vi "Get Switch.vi"(8 "error in (no error)":errorcluster, 10 "switch name":string="A", 11 "MC switch refnum in":refnum<k24>) -> (0 "error out":errorcluster, 2 "state":bool, 3 "MC switch refnum out":refnum<k24>)   [LabVIEW 2019, in "Minicircuit RF Switch Box.lvlib"]
doc: "This function get an individual SPDT state within the switch matrix. The switches are designated A to H, as labeled on the front of the switch matrix.\n\n<b>Note:</b> If the swish matrix does not have a swich connected to the ask position, nothing will append."
uses:
  <instrlib>/LV_Minicircuit_RF_Switch/Minicircuit RF Switch Box.lvlib
  C:/Program Files (x86)/National Instruments/LabVIEW 2019/instr.lib/LV_Minicircuit_RF_Switch/mcl_RF_Switch_Controller_NET45.dll
  mcl_RF_Switch_Controller_NET45.dll
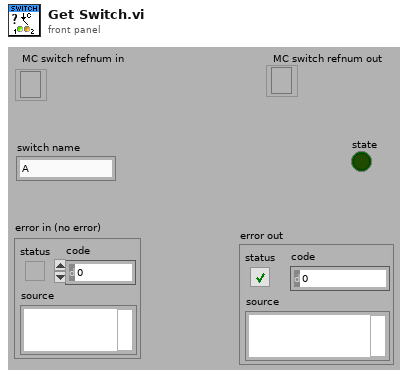
[diagram p1: front panel]
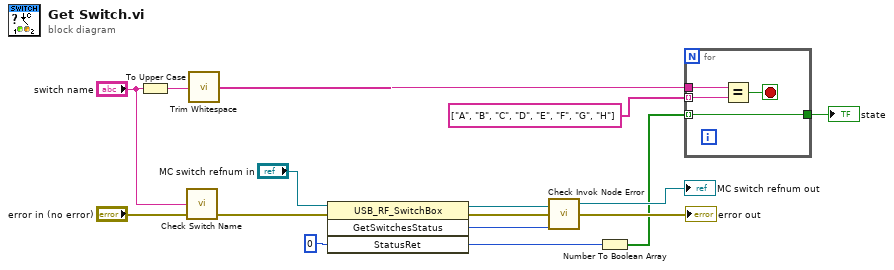
[diagram p0: block diagram]
diagram:
  n1 = To Upper Case(1:"switch name") -> (0:w6:string)
  n2 = call <instrlib>:"Check Switch Name.vi"("error in (no error)"="error in (no error)", "switch name in"="switch name") -> ("error out"=w7:errorcluster)  [unwired: 2 in, 1 out]
  n3 = call <vilib>:"Trim Whitespace.vi"("string"=w6) -> ("trimmed string"=w5:string)  [unwired: 1 in]
  n4 = invoke class="USB_RF_SwitchBox" method="GetSwitchesStatus"(reference="MC switch refnum in", error in=w7, "StatusRet"=0) -> (reference out=w15:refnum<k24>, error out=w14:errorcluster, "GetSwitchesStatus"=w13:i32, "StatusRet"=w9:i32)  [unwired: 1 in]
  n5 = call <instrlib>:"Check Invok Node Error.vi"("Connect"=w13, "error in (no error)"=w14, "MC switch refnum in"=w15) -> ("error out"=→"error out":errorcluster, "MC switch refnum out"=→"MC switch refnum out":refnum<k24>)  [unwired: 1 in]
  n6 = Number To Boolean Array(number=w9) -> (Boolean array=w2:bool[])
  n7 = for {
    tunnel: w5 -> [w20]
    tunnel: string[] ["A", "B", "C", "D", "E", "F", "G", "H"] -> [w19] mode=indexing
    tunnel: [w17] -> w1
    tunnel: w2 -> [w17] mode=indexing
    stop <- w18 stop-if-true
    n8 = Equal?(x=w20, y=w19) -> (x = y?=w18:bool)
  }
  "state" <- w1
